vi "wrap.GetArraySizes.vi"(0 "class.GLue in":refnum<class "class.GLue.lvclass">, 11 "error in (no error)":errorcluster) -> (2 "2DArray":bool, 4 "class.GLue out":refnum<class "class.GLue.lvclass">, 8 "Array Type":i32, 12 "Columns":i32, 14 "Rows":i32, 15 "error out":errorcluster)   [LabVIEW 2014, in "GLue.lvlib" / "class.GLue.lvclass"]
uses:
  class.GLue.lvclass
  class.GLue.lvclass/class.GLue.ctl
  Resources/GLue.dll
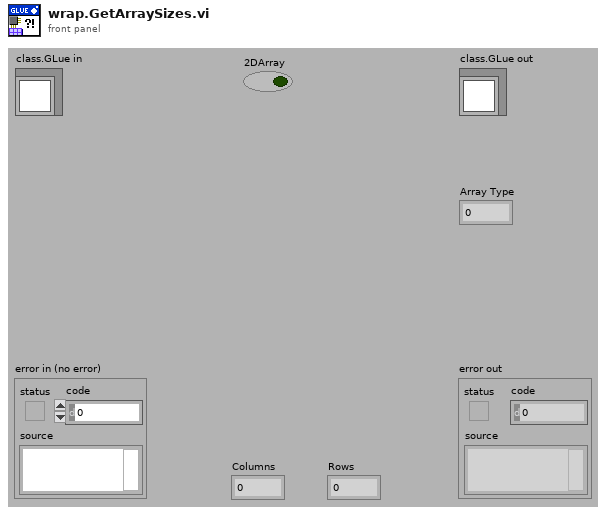
[diagram p1: front panel]
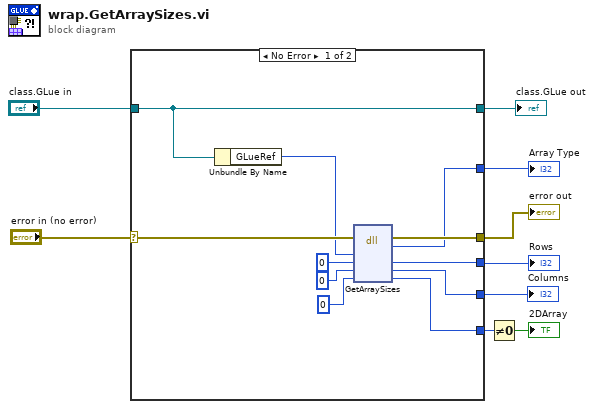
[diagram p0: block diagram]
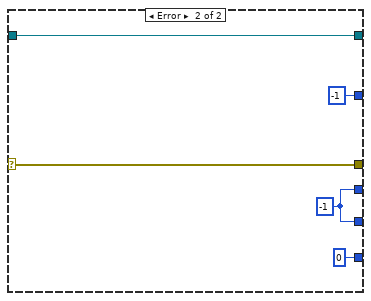
[diagram p2: hidden frame]
diagram:
  n1 = case shown="No Error" "error in (no error)" {
    selector: "error in (no error)" -> [w19 w25]
    tunnel: [w18 w25] -> w8
    tunnel: [w20 w24] -> w6
    tunnel: "class.GLue in" -> [w20 w24]
    tunnel: [w14 w23] -> w4
    tunnel: [w13 w23] -> w3
    tunnel: [w12 -1 ("return type")] -> w5
    tunnel: [w11 0 ("is2D")] -> w1
    frame No Error {
      n2 = Unbundle By Name(w20) -> ("GLueRef"=w17:i64)
      n3 = dll-call lib="C:/Users/Antonie/Documents/work/glue/trunk/Resources/GLue.dll" fn="GetArraySizes"(error in=w19, "MLua"=w17, "Rows"=0, "Columns"=0 ("Rows"), "is2D"=0) -> (error out=w18:errorcluster, "return type"=w12:i32, "Rows"=w14:i32, "Columns"=w13:i32, "is2D"=w11:i32)  [unwired: 3 in, 1 out]
    }
    frame Error {
      w23 = -1 ("TopType")
    }
  }
  "error out" <- w8
  "class.GLue out" <- w6
  "Rows" <- w4
  "Columns" <- w3
  "Array Type" <- w5
  n4 = Not Equal To 0?(x=w1) -> (x != 0?=→"2DArray":bool)
